vi "example.vi"(8 "error in (no error)":errorcluster caption="错误输入（无错误）", 11 "data_in":T4={"table"="分体式气象大风时段", "columns"=["时间", "大风时段开始时间", "大风时段结束时间"], "condition"="", "data_in"={"PW"="123456", "MN"="TEST001", "table输入"="水文气象统计数据", "数据发送次数"=0, "枚举"=enum."上传数据", "type"="000", "因子编码&数据类型"=[{"因子编码"="e01306", "数据类型"="-Starttime="}, {"因子编码"="e01307", "数据类型"="-Endtime="}]}}) -> (0 "error out":errorcluster caption="错误输出", 2 "最新时间":string, 3 "message":string[](array[string]))   [LabVIEW 2016, in "中水三立SQL数据传输.lvlib"]
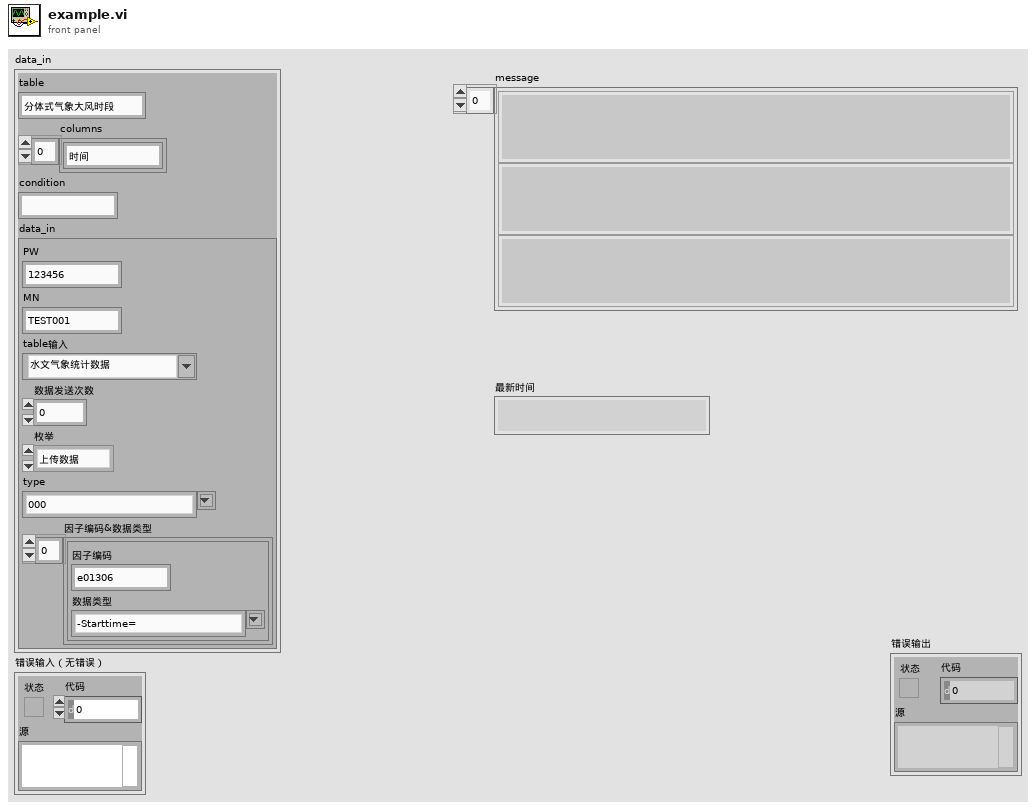
[diagram p1: front panel]
types:
  T1 = typedef "中水三立SQL数据传输.lvlib/data_in.ctl" = cluster{"PW":string, "MN":string, "table输入":T2, "数据发送次数":i32, "枚举":enum16{"返回请求应答", "上传数据", "返回执行结果"}, "type":T3, "因子编码&数据类型":cluster{"因子编码":string, "数据类型":string}[]}
  T2 = typedef "中水三立SQL数据传输.lvlib/table.ctl" = string
  T3 = typedef "中水三立SQL数据传输.lvlib/Type.ctl" = string
  T4 = cluster{"table":string, "columns":string[], "condition":string, "data_in":T1}
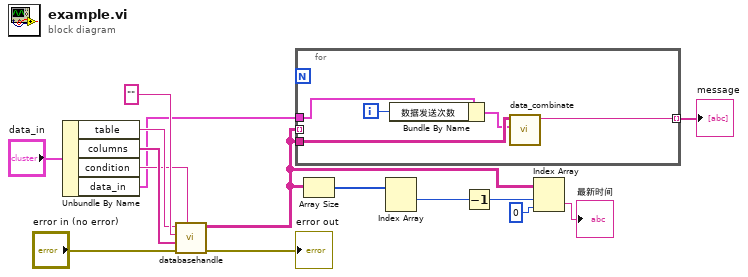
[diagram p0: block diagram]
diagram:
  n1 = Unbundle By Name("data_in") -> ("table"=w14:string, "columns"=w13:string[], "condition"=w10:string, "data_in"=w9:T1)
  n2 = call "databasehandle.vi"("condition"=w10, "error in (no error)"="error in (no error)", "columns"=w13, "password"="", "table"=w14) -> ("error out"=→"error out":errorcluster, "data"=w6:string[][])  [unwired: 5 in]
  n3 = for {
    tunnel: w6 -> [w18]
    tunnel: w9 -> [w20]
    tunnel: w6 -> [_] mode=indexing
    tunnel: [w17] -> w12 mode=indexing
    i -> [w19]
    n4 = Bundle By Name(cluster=w20, "数据发送次数"=w19) -> (w16:T1)
    n5 = call "data_combinate.vi"("data_in"=w16, "data"=w18) -> ("message"=w17:string)  [unwired: 8 in, 1 out]
  }
  "message" <- w12
  n6 = Array Size(array=w6) -> (size(s)=w5:i32[])
  n7 = Index Array(array=w5) -> (element #1=w4:i32)  [unwired: 2 in, 1 out]
  n8 = Decrement(x=w4) -> (x-1=w3:i32)
  n9 = Index Array(array=w6, index (row)=w3, index (col)=0 ("禁用的索引 (列)")) -> (element=→"最新时间":string)
